vi "GetTimeInSecFromArr.vi"(10 "Current step":i32, 11 "all rows":i64[][](array[numeric])) -> (3 "Time in sec":dbl)   [LabVIEW 2017]
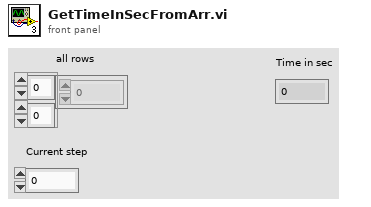
[diagram p1: front panel]
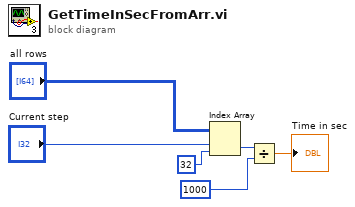
[diagram p0: block diagram]
diagram:
  n1 = Index Array(array="all rows", index (row)="Current step", index (col)=32 ("disabled index (col)")) -> (element=w5:i64)
  n2 = Divide(x=w5, y=i64 1000) -> (x/y=→"Time in sec":dbl)
